vi "Contour Finding Test.vi"() -> ()   [LabVIEW 2011]
uses:
  <vilib>/vision/NI_Vision_Development_Module.lvlib
  <vilib>/Platform/TimedLoop/XDataNode/XDataNode.xnode
  <vilib>/Platform/TimedLoop/XDataNode/nitl_modes.ctl
  <vilib>/Platform/TimedLoop/XDataNode/XDNodeRunTimeDep.lvlib
  <vilib>/Platform/TimedLoop/XDataNode/wakeup.ctl
  <vilib>/Platform/TimedLoop/XDataNode/timing_clust.ctl
  <vilib>/vision/Analysis.llb/IMAQ ExtractCurvesCurve.ctl
  <vilib>/vision/Pattern Matching.llb/IMAQ Curve Parameters.ctl
panel:
  in  "Width":u32=8
  in  "stop":bool
  in  "Curve Parameters":T1={"Extraction Mode"=0, "Edge Threshold"=7, "Edge Filter Size"=1, "Min Length"=25, "Row Search Step Size"=15, "Col Search Step Size"=15, "Max Endpoint Gap"=10, "Closed"=FALSE, "Subpixel"=FALSE} {"Extraction Mode" items=["Normal", "Uniform Regions"]; "Edge Filter Size" items=["Fine", "Normal", "Contour Tracing"]; "Max Endpoint Gap" min=0; "Col Search Step Size" min=1 max=255 step=1; "Row Search Step Size" min=1 max=255 step=1; "Min Length" min=0; "Edge Threshold" min=1 max=350 step=1}
  out "Original image":T2(plugin-control)
  out "Curves":T3[](array[typedef]) {"Points"."Y" format="%.2f"; "Points"."X" format="%.2f"}
  out "Thresholded":T2(plugin-control)
  in  "Range":cluster{"Lower value":sgl, "Upper value":sgl}={"Lower value"=10.0, "Upper value"=32768.0} {"Upper value" format="%.2f"; "Lower value" format="%.2f"}
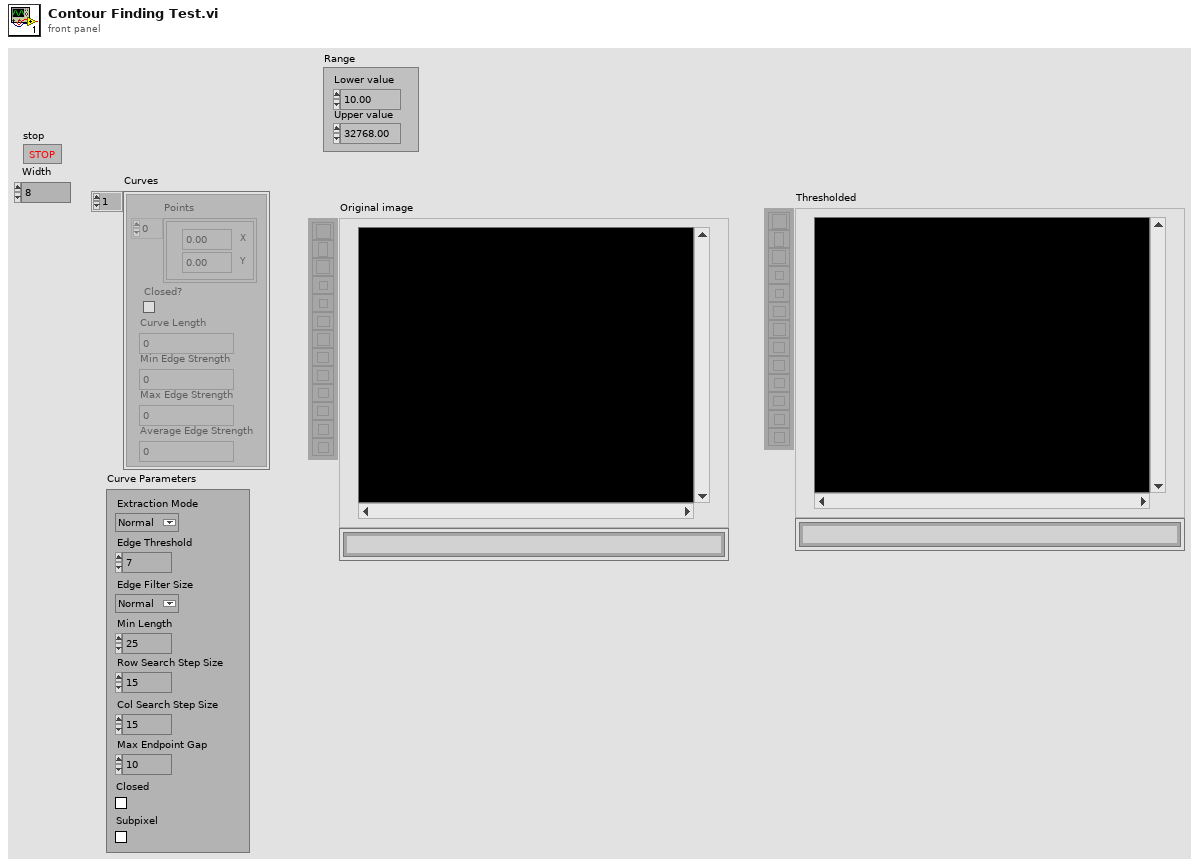
[diagram p1: front panel]
types:
  T1 = typedef "IMAQ Curve Parameters.ctl" = cluster{"Extraction Mode":u32, "Edge Threshold":i32, "Edge Filter Size":u32, "Min Length":i32, "Row Search Step Size":i32, "Col Search Step Size":i32, "Max Endpoint Gap":i32, "Closed":bool, "Subpixel":bool}
  T2 = typedef "IMAQ Image.ctl" = refnum<image>
  T3 = typedef "IMAQ ExtractCurvesCurve.ctl" = cluster{"Points":cluster{"X":dbl, "Y":dbl}[], "Closed?":bool, "Curve Length":dbl, "Min Edge Strength":dbl, "Max Edge Strength":dbl, "Average Edge Strength":dbl}
  T4 = typedef "Image Type" = u32
  T5 = typedef "XDNodeRunTimeDep.lvlib/timing_clust.ctl" = cluster{"Expected End [f-1]":u64, "Actual End [f-1]":u64, "Finished Late? [f-1]":bool, "Expected End [i-1]":u64, "Actual End [i-1]":u64, "Finished Late? [i-1]":bool, "Expected Start [i]":u64, "Actual Start [i]":u64, "Expected Start [f]":u64, "Actual Start [f]":u64, "Source Name":string, "Structure Name":string, "Period":i64, "Deadline":i64, "Offset":i64, "Start":i64, "Priority":i32, "Timeout":i32, "Mode":T6, "Wakeup Reason":T7, "Error":errorcluster, "Source Type":string, "Secondary Source Type":string, "Global End Time":u64, "Global Start Time":u64, "Frame Duration":u64, "Iteration Duration":u64, "Assigned CPU":i32, "I/O Scan Engine Mode":u32}
  T6 = typedef "XDNodeRunTimeDep.lvlib/nitl_modes.ctl" = enum32{"No Change", "Process missed periods, maintain original phase", "Discard missed periods, maintain original phase", "Process missed periods, ignore original phase", "Discard missed periods, ignore original phase"}
  T7 = typedef "XDNodeRunTimeDep.lvlib/wakeup.ctl" = enum32{"Normal", "Aborted", "Asynchronous wakeup", "Timing source error", "Timed loop error", "Timeout"}
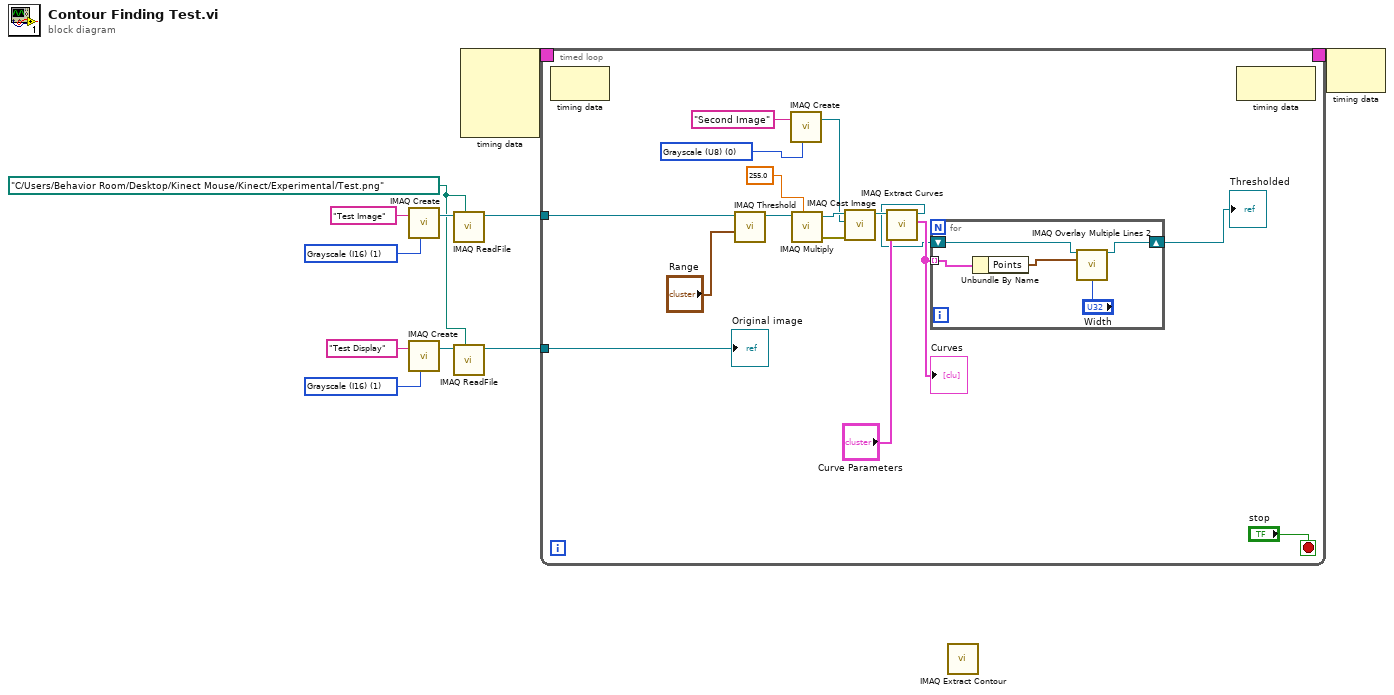
[diagram p0: block diagram]
diagram:
  w7 = T4 1 items=["Grayscale (U8)", "Grayscale (I16)", "Grayscale (SGL)", "Complex (CSG)", "RGB (U32)", "HSL (U32)", "RGB (U64)", "Grayscale (U16)"] ("Image Type")
  w3 = path "C:/Users/Behavior Room/Desktop/Kinect Mouse/Kinect/Experimental/Test.png" ("File Path")
  w11 = T4 1 items=["Grayscale (U8)", "Grayscale (I16)", "Grayscale (SGL)", "Complex (CSG)", "RGB (U32)", "HSL (U32)", "RGB (U64)", "Grayscale (U16)"] ("Image Type")
  n1 = call "IMAQ Create"("Image Name"="Test Image", "Image Type"=w11) -> ("New Image"=w9:T2)  [unwired: 3 in, 1 out]
  n2 = call "IMAQ Create"("Image Name"="Test Display", "Image Type"=w7) -> ("New Image"=w5:T2)  [unwired: 3 in, 1 out]
  n3 = call "IMAQ ReadFile"("File Path"=w3, "Image"=w9) -> ("Image Out"=w8:T2)  [unwired: 5 in, 4 out]
  n4 = call "IMAQ ReadFile"("File Path"=w3, "Image"=w5) -> ("Image Out"=w4:T2)  [unwired: 5 in, 4 out]
  n5 = node-c288() -> (w2:T5)  [unwired: 4 in]
  n6 = timed-loop {
    tunnel: w8 -> [w20]
    tunnel: w4 -> [w19]
    timing: w2 -> [_]
    timing-out: [_] -> w1
    stop <- "stop" stop-if-true
    w22 = T4 0 items=["Grayscale (U8)", "Grayscale (I16)", "Grayscale (SGL)", "Complex (CSG)", "RGB (U32)", "HSL (U32)", "RGB (U64)", "Grayscale (U16)"] ("Image Type")
    n7 = node-c288() -> ()  [unwired: 1 in, 1 out]
    n8 = call "IMAQ Threshold"("Range"="Range", "Image Src"=w20) -> ("Image Dst Out"=w26:T2)  [unwired: 8 in, 1 out]
    n9 = call "IMAQ Create"("Image Name"="Second Image", "Image Type"=w22) -> ("New Image"=w21:T2)  [unwired: 3 in, 1 out]
    n10 = call "IMAQ Multiply"("Image Src A"=w26, "Constant"=sgl 255.0) -> ("Image Dst Out"=w24:T2, "error out"=w25:errorcluster)  [unwired: 5 in]
    n11 = call "IMAQ Cast Image"("error in (no error)"=w25, "Image Dst"=w21, "Image Src"=w24) -> ("Image Dst Out"=w17:T2)  [unwired: 7 in, 1 out]
    n12 = call "IMAQ Extract Curves"("Curve Parameters"="Curve Parameters", "Image"=w17) -> ("Curves"=w16:T3[], "Image (dup)"=w13:T2)  [unwired: 7 in, 1 out]
    "Curves" <- w16
    n13 = for {
      tunnel: w16 -> [w34] mode=indexing
      shift-right: [w30] -> w12
      shift-left: w13 -> [w32]
      n14 = Unbundle By Name(w34) -> ("Points"=w33:cluster{"X":dbl, "Y":dbl}[])
      n15 = call "IMAQ Overlay Multiple Lines 2"("Image"=w32, "Line End Points"=w33, "Width"="Width") -> ("Image Out"=w30:T2)  [unwired: 11 in, 1 out]
    }
    "Thresholded" <- w12
    n16 = node-c288() -> ()  [unwired: 1 in, 1 out]
    "Original image" <- w19
  }
  n17 = call "IMAQ Extract Contour"() -> ()  [unwired: 11 in, 5 out]
  n18 = node-c288(w1) -> ()  [unwired: 1 out]
